vi "Check Channel.vi"(8 "Error In":errorcluster) -> (0 "Error Out":errorcluster)   [LabVIEW 2011, in "LVH-LINX.lvlib" / "Device.lvlib"]
uses:
  Device.lvlib
  Type Defs/Peripheral.ctl
  LVH-LINX.lvlib
panel:
  in  "Peripheral":T1
  in  "Channel Number":u8
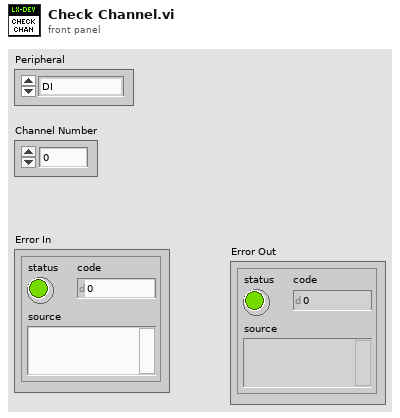
[diagram p1: front panel]
types:
  T1 = typedef "LVH-LINX.lvlib/Peripheral.ctl" = enum8{"DI", "DO", "AI", "AO", "PWM", "QE", "UART", "I2C", "SPI", "CAN"}
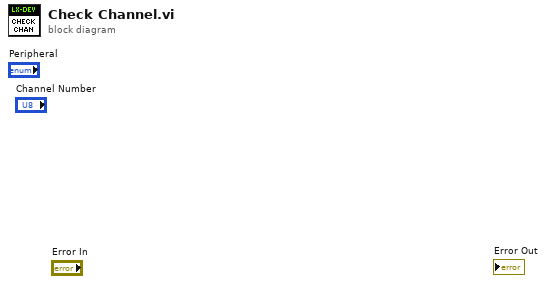
[diagram p0: block diagram]
diagram:
